vi "Letter to ASCII Array.vi"(8 "error in (no error)":errorcluster, 11 "Input String":string) -> (0 "error out":errorcluster, 3 "String to ASCII Array":u8[](array[numeric]))   [LabVIEW 2018]
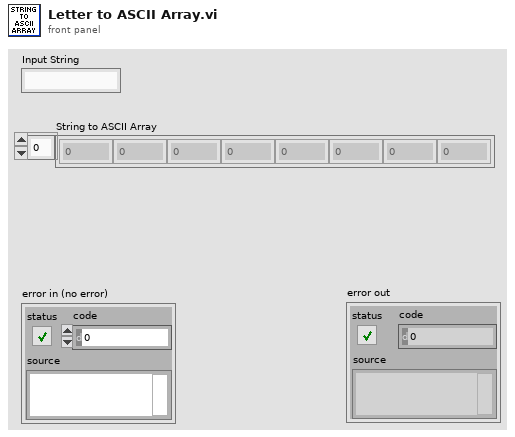
[diagram p1: front panel]
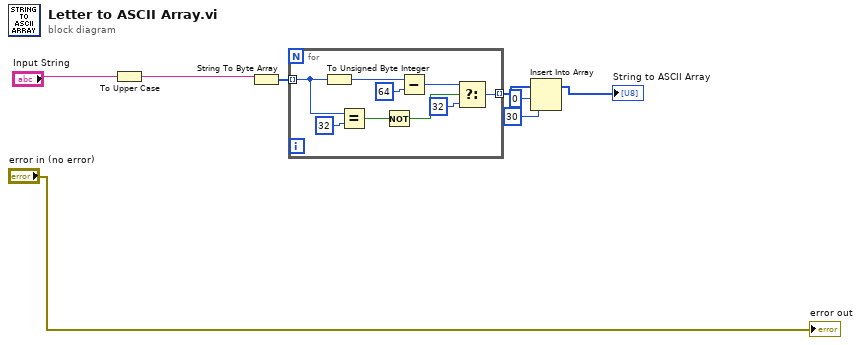
[diagram p0: block diagram]
diagram:
  n1 = To Upper Case(1:"Input String") -> (0:w5:string)
  n2 = String To Byte Array(string=w5) -> (unsigned byte array=w8:u8[])
  n3 = for {
    tunnel: w8 -> [w12] mode=indexing
    tunnel: [w13] -> w4 mode=indexing
    n4 = To Unsigned Byte Integer(number=w12) -> (unsigned 8bit integer=w17:u8)
    n5 = Equal?(x=w12, y=u8 32) -> (x = y?=w10:bool)
    n6 = Not(x=w10) -> (.not. x?=w9:bool)
    n7 = Subtract(x=w17, y=u8 64) -> (x-y=w14:u8)
    n8 = Select(t=w14, s=w9, f=u8 32) -> (s? t:f=w13:u8)
  }
  n9 = Insert Into Array(array=w4, index=0, new element=u8 30 ("new element/subarray")) -> (→"String to ASCII Array":u8[])
  "error out" <- "error in (no error)"
